vi "Identify.vi"(8 "error in (no error)":errorcluster, 11 "Input Power MSMT In":refnum<class "Input Power Measurement.lvclass">) -> (0 "error out":errorcluster, 2 "Plugin is Valid":bool, 3 "Input Power MSMT Out":refnum<class "Input Power Measurement.lvclass">)   [LabVIEW 2018, in "Input Power Measurement.lvlib" / "Input Power Measurement.lvclass"]
uses:
  Input Power Measurement.lvclass
  C:/Sequence Automation/Plugins/Measurement Interface.lvlibp/Measurement Interface.lvclass
  Plugins/Measurement Interface.lvlibp/Private Methods/Measurement Definition Entry/Read Measurement Definition Entry.vi
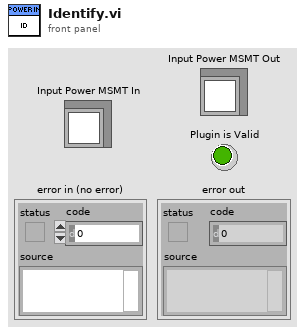
[diagram p1: front panel]
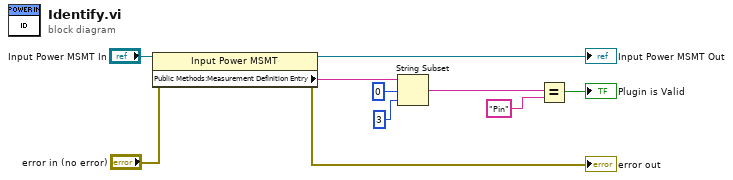
[diagram p0: block diagram]
diagram:
  n1 = property class="Input Power MSMT"(reference="Input Power MSMT In", error in="error in (no error)") -> (reference out=→"Input Power MSMT Out":refnum<class "Input Power Measurement.lvclass">, error out=→"error out":errorcluster, "Public Methods:Measurement Definition Entry"=w6:string)
  n2 = String Subset(string=w6, offset (0)=0, length (rest)=3 ("length (rest)")) -> (substring=w3:string)
  n3 = Equal?(x=w3, y="Pin") -> (x = y?=→"Plugin is Valid":bool)
